vi "CurrentValueUI.vi"() -> ()   [LabVIEW 2016]
uses:
  <vilib>/Utility/error.llb/DialogType.ctl
  <vilib>/Utility/miscctls.llb/LVRowAndColumnTypeDef.ctl
  Architecture/Queue Management/ARC_Queue Create_Single.vi
  Architecture/Queue Management/ARC_Queue Valid.vi
  Architecture/Queue Management/ARC_Queue Remove Element.vi
  MainUI/Config Display Font Size.vi
  Architecture/Queue Management/ARC_Queue Insert Element.vi
  Architecture/Queue Management/ARC_Queue Destroy_Single.vi
panel:
  in  "CurrentValues":i32(listbox)
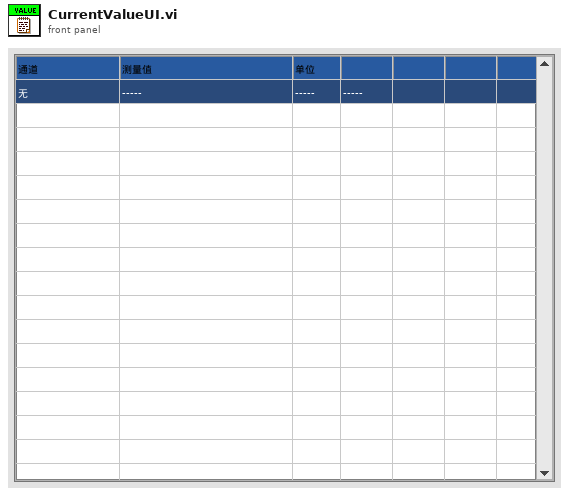
[diagram p1: front panel]
types:
  T1 = cluster{"error":errorcluster, "Event":string, "Data":variant, "Q_Local":string, "ListRef":refnum<vi>, "Q_Caller":string}
  T2 = typedef "LVRowAndColumnTypeDef.ctl" = cluster{"Row":i32, "Column":i32}
  T3 = typedef "DialogType.ctl" = u16
  T4 = cluster{"Channel Font Size":u32, "Channel Value Font Size":u32, "Unit Font Size":u32, "Row Font Size":u32, "Display Precision":u32}
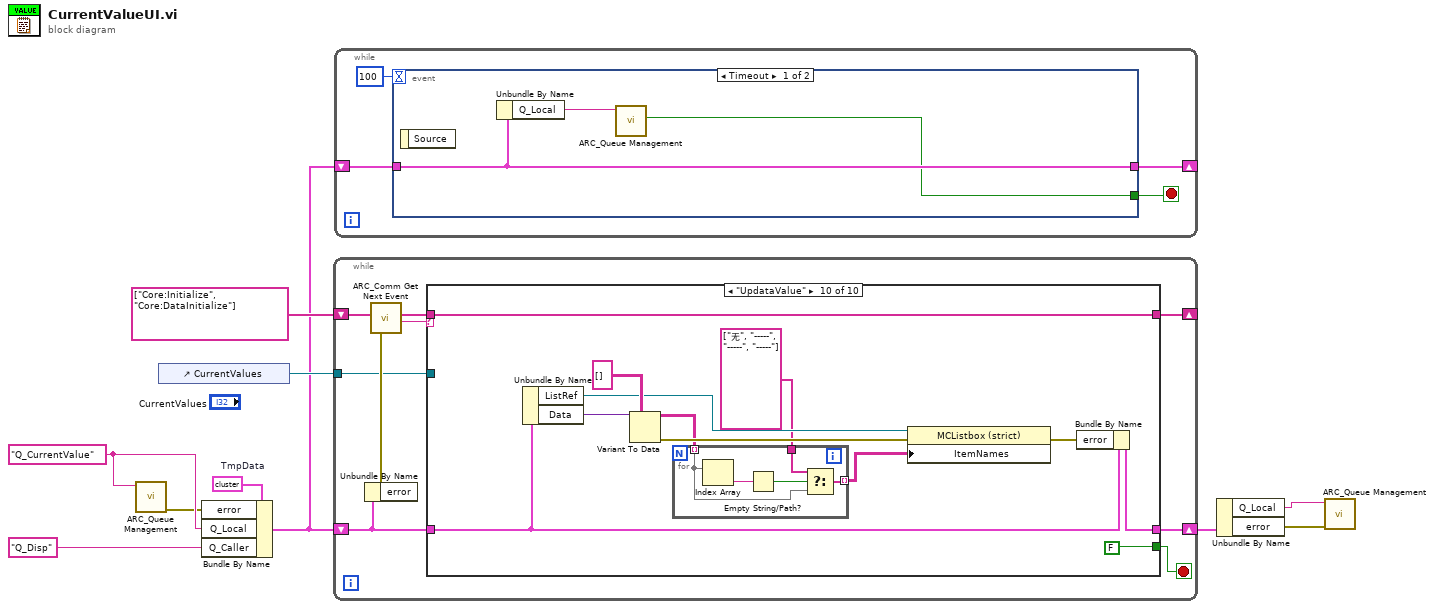
[diagram p0: block diagram]
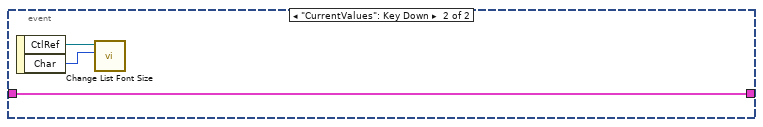
[diagram p2: hidden frame]
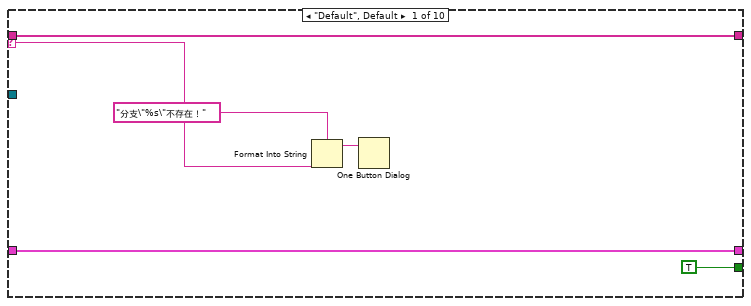
[diagram p3: hidden frame]
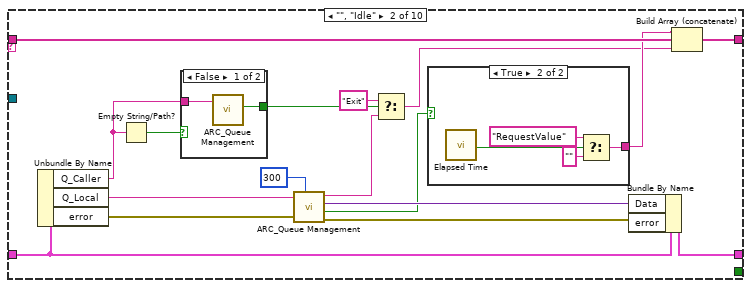
[diagram p4: hidden frame]
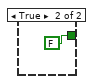
[diagram p5: hidden frame]
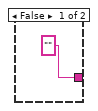
[diagram p6: hidden frame]
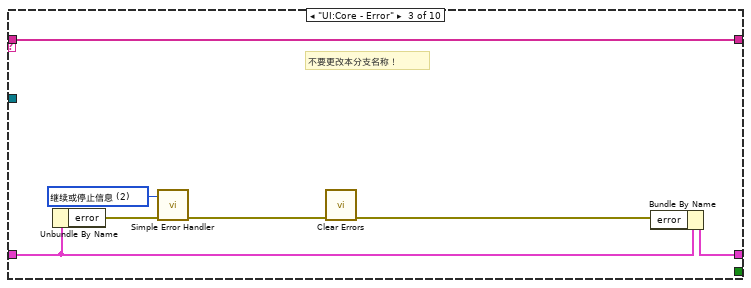
[diagram p7: hidden frame]
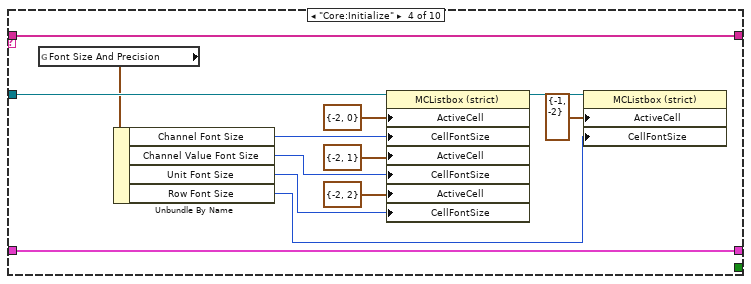
[diagram p8: hidden frame]
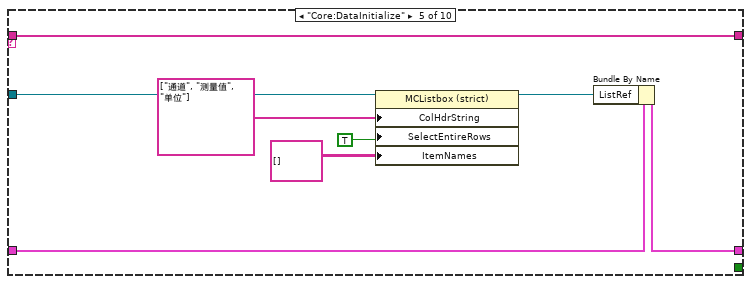
[diagram p9: hidden frame]
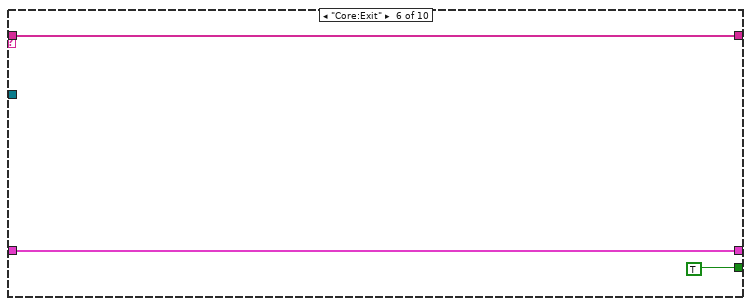
[diagram p10: hidden frame]
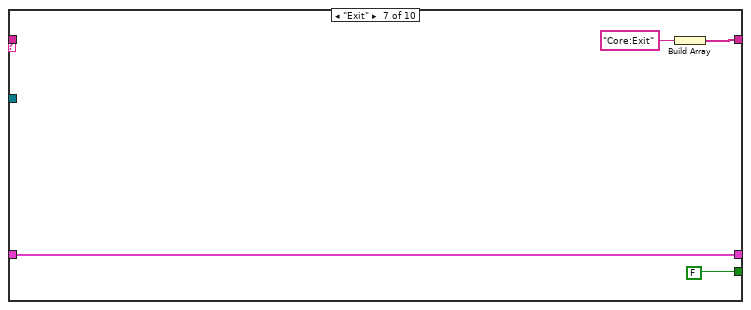
[diagram p11: hidden frame]
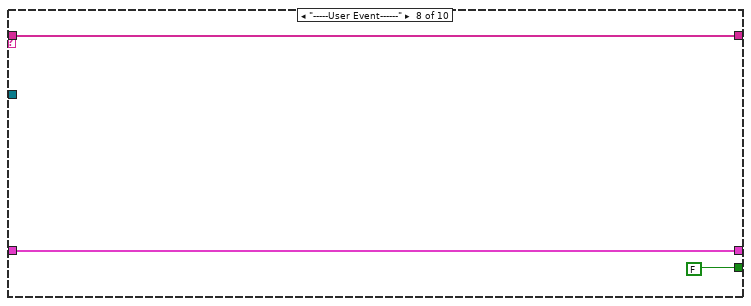
[diagram p12: hidden frame]
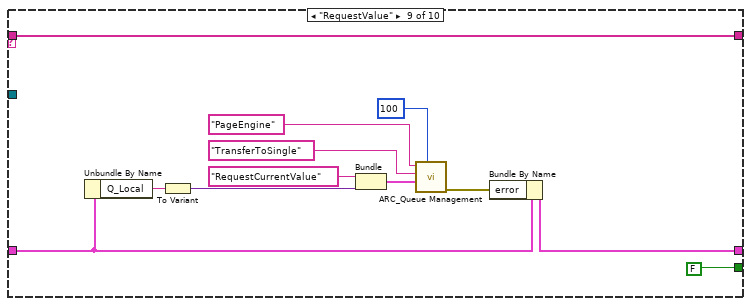
[diagram p13: hidden frame]
diagram:
  w8 = T1 {"error"={"status"=FALSE, "code"=0, "source"=""}, "Event"="", "Data"=variant, "Q_Local"="", "ListRef"=refnum, "Q_Caller"=""}  # TmpData
  w7 = "Q_CurrentValue" ("QueueName")
  n1 = call-poly "ARC_Queue Management.vi"("Queue Name"=w7) -> ("error out"=w5:errorcluster)  [unwired: 8 in, 2 out]
  n2 = control-ref of="CurrentValues"() -> (w3:refnum<vi>)
  n3 = Bundle By Name(cluster=w8, "error"=w5, "Q_Local"=w7, "Q_Caller"="Q_Disp") -> (w1:T1)
  n4 = while {
    shift-right: [w15] -> w9
    shift-left: w1 -> [w16]
    shift-right: [w14] -> _
    shift-left: string[] ["Core:Initialize", "Core:DataInitialize"] ("event queue out") -> [w11]
    tunnel: w3 -> [w13]
    stop <- w18 stop-if-true
    n5 = Unbundle By Name(w16) -> ("error"=w17:errorcluster)
    n6 = call "ARC_Comm Get Next Event.vi"("error in (no error)"=w17, "event queue in"=w11) -> ("next event"=w12:string, "event queue out"=w19:string[])  [unwired: 4 in, 1 out]
    n7 = case shown="\"UpdataValue\"" w12 {
      selector: w12 -> [w23 _ _ _ _ _ _ _ _ _]
      tunnel: w19 -> [w24 w30 w57 w58 w78 w79 _ w86 w99 w111]
      tunnel: [TRUE _ _ _ _ TRUE FALSE FALSE FALSE FALSE] -> w18
      tunnel: w16 -> [w25 w39 w53 w70 w77 w80 w84 w87 w92 w105]
      tunnel: [w25 w41 w52 w70 w76 w80 w84 w87 w90 w104] -> w15
      tunnel: [w24 w29 w57 w58 w78 w79 w82 w86 w99 w111] -> w14
      tunnel: w13 -> [_ _ _ w69 w71 _ _ _ _ _]
      frame "Default", Default {
        n8 = Format Into String(format string="分支\"%s\"不存在！" ("格式字符串"), w23) -> (resulting string=w22:string)  [unwired: 2 in, 1 out]
        n9 = One Button Dialog(message=w22) -> ()  [unwired: 1 in, 1 out]
      }
      frame "", "Idle" {
        n10 = Unbundle By Name(w39) -> ("Q_Caller"=w34:string, "Q_Local"=w38:string, "error"=w37:errorcluster)
        n11 = Empty String/Path?(string/path=w34) -> (empty?=w35:bool)
        n12 = case shown="False" w35 {
          tunnel: [w43 FALSE ("Not Exist?")] -> w33
          tunnel: w34 -> [w44 _]
          frame False {
            n13 = call-poly "ARC_Queue Management.vi"("Queue Name(unamed)"=w44) -> ("Not Exist?"=w43:bool)  [unwired: 8 in, 2 out]
          }
          frame True {
          }
        }
        n14 = call-poly "ARC_Queue Management.vi"("Time out(-1)_queue out"=300 ("Time out(-1)"), "error in (no error)"=w37, "Queue Name(unamed)"=w38) -> ("error out"=w42:errorcluster, "timed out"=w36:bool, "Data"=w40:variant, "Event"=w31:string)  [unwired: 5 in]
        n15 = Select(t="Exit" ("Event"), s=w33, f=w31) -> (s? t:f=w27:string)
        n16 = case shown="True" w36 {
          tunnel: ["" ("t") w48] -> w28
          frame False {
          }
          frame True {
            n17 = call "Elapsed Time"() -> ("Time has Elapsed"=w47:bool)  [unwired: 12 in, 7 out]
            n18 = Select(t="RequestValue", s=w47, f="") -> (s? t:f=w48:string)
          }
        }
        n19 = Bundle By Name(cluster=w39, "Data"=w40, "error"=w42) -> (w41:T1)
        n20 = Build Array (concatenate)(w28, w30, w27) -> (w29:string[])
      }
      frame "UI:Core - Error" {
        w51 = T3 2 items=["无对话框", "确定信息", "继续或停止信息", "确定信息＋警告", "继续/停止+警告"] ("type of dialog (OK msg:1)")
        # "不要更改本分支名称！"
        n21 = Unbundle By Name(w53) -> ("error"=w54:errorcluster)
        n22 = call <vilib>:"Simple Error Handler.vi"("type of dialog (OK msg:1)"=w51, "error in (no error)"=w54) -> ("error out"=w55:errorcluster)  [unwired: 3 in, 4 out]
        n23 = call <vilib>:"Clear Errors.vi"("error in (no error)"=w55) -> ("error out"=w56:errorcluster)  [unwired: 5 in, 1 out]
        n24 = Bundle By Name(cluster=w53, "error"=w56) -> (w52:T1)
      }
      frame "Core:Initialize" {
        n25 = global read "Config Display Font Size.vi" "Font Size And Precision"() -> (w63:T4)
        n26 = Unbundle By Name(w63) -> ("Channel Font Size"=w62:u32, "Channel Value Font Size"=w61:u32, "Unit Font Size"=w60:u32, "Row Font Size"=w59:u32)
        n27 = property class="MCListbox (strict)"(reference=w69, "ActiveCell"=T2 {"Row"=-2, "Column"=0} ("活动单元格:活动单元格"), "CellFontSize"=w62, "ActiveCell"=T2 {"Row"=-2, "Column"=1} ("活动单元格:活动单元格"), "CellFontSize"=w61, "ActiveCell"=T2 {"Row"=-2, "Column"=2} ("活动单元格:活动单元格"), "CellFontSize"=w60) -> (reference out=w65:refnum<vi>)  [unwired: 1 in, 1 out]
        n28 = property class="MCListbox (strict)"(reference=w65, "ActiveCell"=T2 {"Row"=-1, "Column"=-2} ("活动单元格:活动单元格"), "CellFontSize"=w59) -> ()  [unwired: 1 in, 2 out]
      }
      frame "Core:DataInitialize" {
        n29 = property class="MCListbox (strict)"(reference=w71, "ColHdrString"=string[] ["通道", "测量值", "单位"] ("Column Header Strings[]"), "SelectEntireRows"=TRUE ("自动调整行高"), "ItemNames"=string[][] [] ("项名")) -> (reference out=w75:refnum<vi>)  [unwired: 1 in, 1 out]
        n30 = Bundle By Name(cluster=w77, "ListRef"=w75) -> (w76:T1)
      }
      frame "Core:Exit" {
      }
      frame "Exit" {
        n31 = Build Array("Core:Exit" ("Remaining States")) -> (w82:string[])
      }
      frame "-----User Event------" {
      }
      frame "RequestValue" {
        n32 = Unbundle By Name(w92) -> ("Q_Local"=w94:string)
        n33 = To Variant(anything=w94) -> (Variant=w93:variant)
        n34 = Bundle("RequestCurrentValue", "Variant"=w93) -> (w95:cluster{string, "Variant":variant})  [unwired: 1 in]
        n35 = call-poly "ARC_Queue Management.vi"("Time out(-1)_queue in"=100, "Data"=w95, "Event"="TransferToSingle", "Queue Name(unamed)"="PageEngine" ("QueueName")) -> ("error out"=w91:errorcluster)  [unwired: 6 in, 1 out]
        n36 = Bundle By Name(cluster=w92, "error"=w91) -> (w90:T1)
      }
      frame "UpdataValue" {
        n37 = Unbundle By Name(w105) -> ("ListRef"=w108:refnum<vi>, "Data"=w110:variant)
        n38 = Variant To Data(type=string[][] [], Variant=w110) -> (data=w103:string[][], error out=w107:errorcluster)  [unwired: 1 in]
        n39 = for {
          tunnel: w103 -> [w115] mode=indexing
          tunnel: [w114] -> w102 mode=indexing
          tunnel: string[] ["无", "-----", "-----", "-----"] -> [w113]
          n40 = Index Array(array=w115) -> (element=w117:string)  [unwired: 1 in]
          n41 = Empty String/Path?(string/path=w117) -> (empty?=w116:bool)
          n42 = Select(t=w113, s=w116, f=w115) -> (s? t:f=w114:string[])
        }
        n43 = property class="MCListbox (strict)"(reference=w108, error in=w107, "ItemNames"=w102) -> (error out=w106:errorcluster)  [unwired: 1 out]
        n44 = Bundle By Name(cluster=w105, "error"=w106) -> (w104:T1)
      }
    }
  }
  n45 = while {
    shift-right: [w119] -> _
    shift-left: w1 -> [w120]
    stop <- w118 stop-if-true
    n46 = event shown="[0] Timeout" {
      selector: _ -> [_ _]
      dyn-events: _ -> [_ _]
      timeout: 100 -> [_ _]
      tunnel: w120 -> [w124 w127]
      tunnel: [w124 w127] -> w119
      tunnel: [w122 _] -> w118
      event Timeout {
        n47 = event-data() -> ()  [unwired: 1 in, 1 out]
        n48 = Unbundle By Name(w124) -> ("Q_Local"=w123:string)
        n49 = call-poly "ARC_Queue Management.vi"("Queue Name(unamed)"=w123) -> ("Not Exist?"=w122:bool)  [unwired: 8 in, 2 out]
      }
      event "CurrentValues": Key Down {
        n50 = event-data() -> ("CtlRef"=w126:refnum<vi>, "Char"=w125:i16)  [unwired: 1 in]
        n51 = call "Change List Font Size.vi"("Char"=w125, "MulticolumnListbox in"=w126) -> ()  [unwired: 9 in, 1 out]
      }
    }
  }
  n52 = Unbundle By Name(w9) -> ("Q_Local"=w6:string, "error"=w10:errorcluster)
  n53 = call-poly "ARC_Queue Management.vi"("error in (no error)"=w10, "Queue Name(unamed)"=w6) -> ()  [unwired: 7 in, 3 out]
